vi "4.4.vi"(0 "温度":dbl) -> ()   [LabVIEW 2017]
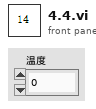
[diagram p1: front panel]
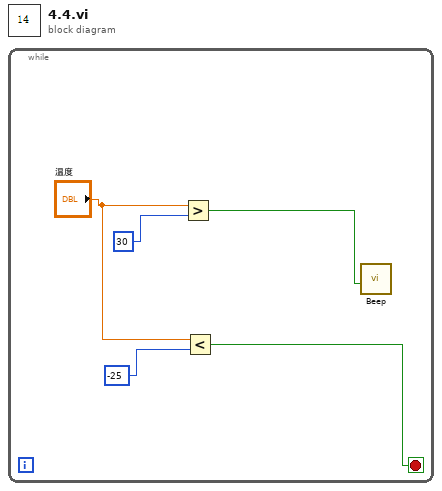
[diagram p0: block diagram]
diagram:
  n1 = while {
    stop <- w1 stop-if-true
    n2 = Greater?(x="温度", y=30) -> (0:w4:bool)
    n3 = Less?(x="温度", y=-25) -> (x < y?=w1:bool)
    n4 = call <vilib>:"Beep.vi"("use system alert? (T)"=w4) -> ()  [unwired: 11 in]
  }
